vi "HH Status.vi"(9 "FIFO Indexes":T1[](array[typedef]), 10 "HH Status":T2[](array[typedef]) {"Current [A]" format="%#_6p"; "On Avg [A]" format="%#_6p"; "Period Avg [A]" format="%#_6p"; "Period Max [A]" format="%#_6p"; "Period Min [A]" format="%#_6p"}, 11 "Device Outputs in":dbl[](array[numeric])) -> (3 "Device Outputs out":dbl[](array[numeric]))   [LabVIEW 2016, in "DCM Engine.lvlib"]
uses:
  DCM Engine.lvlib
  Built/DCM Classes Packed/Pharlap/C/DCM-Classes.lvlibp/DCM/HH/RT/Status.ctl
  Shared/Types/HH Status Indexes.ctl
  DCM Shared.lvlib
  Built/DCM Classes Packed/Pharlap/C/DCM-Classes.lvlibp/DCM/HH/RT/DCM - RT - HH.lvlib
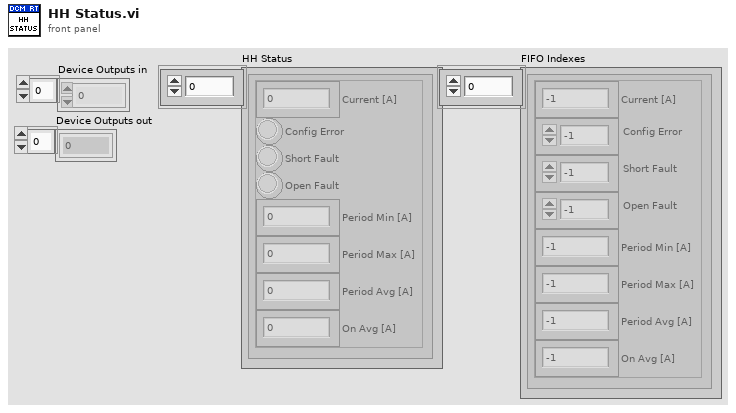
[diagram p1: front panel]
types:
  T1 = typedef "DCM Shared.lvlib/HH Status Indexes.ctl" = cluster{"Current [A]":i32, "Config Error":i32, "Short Fault":i32, "Open Fault":i32, "Period Min [A]":i32, "Period Max [A]":i32, "Period Avg [A]":i32, "On Avg [A]":i32}
  T2 = typedef "DCM-Classes.lvlibp/DCM - RT - HH.lvlib/Status.ctl" = cluster{"Current [A]":sgl, "Config Error":bool, "Short Fault":bool, "Open Fault":bool, "Period Min [A]":sgl, "Period Max [A]":sgl, "Period Avg [A]":sgl, "On Avg [A]":sgl}
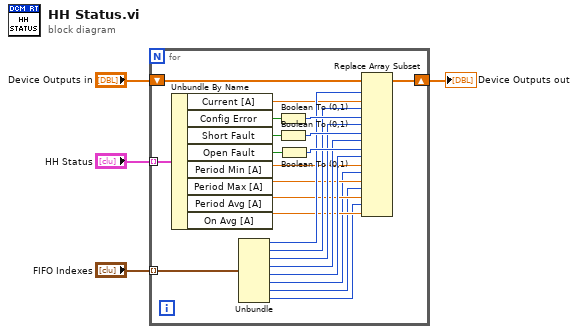
[diagram p0: block diagram]
diagram:
  n1 = for {
    tunnel: "HH Status" -> [w25] mode=indexing
    tunnel: "FIFO Indexes" -> [w18] mode=indexing
    shift-right: [w26] -> w3
    shift-left: "Device Outputs in" -> [w27]
    n2 = Unbundle By Name(w25) -> ("Current [A]"=w12:sgl, "Config Error"=w24:bool, "Short Fault"=w23:bool, "Open Fault"=w22:bool, "Period Min [A]"=w11:sgl, "Period Max [A]"=w10:sgl, "Period Avg [A]"=w9:sgl, "On Avg [A]"=w8:sgl)
    n3 = Unbundle(w18) -> ("Current [A]"=w17:i32, "Config Error"=w16:i32, "Short Fault"=w15:i32, "Open Fault"=w14:i32, "Period Min [A]"=w13:i32, "Period Max [A]"=w7:i32, "Period Avg [A]"=w6:i32, "On Avg [A]"=w5:i32)
    n4 = Boolean To (0,1)(Boolean=w24) -> (0, 1=w21:i16)
    n5 = Boolean To (0,1)(Boolean=w23) -> (0, 1=w20:i16)
    n6 = Boolean To (0,1)(Boolean=w22) -> (0, 1=w19:i16)
    n7 = Replace Array Subset(array=w27, new element #1=w12, index #1=w17, new element #2=w21, index #2=w16, new element #3=w20, index #3=w15, new element #4=w19, index #4=w14, new element #5=w11, index #5=w13, new element #6=w10, index #6=w7, new element #7=w9, index #7=w6, new element #8=w8, index #8=w5) -> (w26:dbl[])
  }
  "Device Outputs out" <- w3
